vi "Triggers-Start.vi"(7 "Setup/Logging queue element":T1={"Imaging Protocol"=enum."Live Imaging", "Number of Trials"=0, "Frame Size"=512, "# Averaged frames"=0, "Dwell time (us)"=0.0, "Index of Z-plane"=0, "Timelapse?"=FALSE, "Logging process is active"=FALSE, "Speed logging enabled"=FALSE, "tdms file ref"=refnum, "path"=path "", "Trial Number"=0, "Expected # points acquired"=FALSE, "Manually stopped"=FALSE, "Ch0 data"=[], "Ch1 data"=[], "Last trial"=FALSE, "Points acquired"={"Ch0 last trial"=0, "Ch1 last trial"=0, "All trials"=0}} {"Frame Size" items=["100X100"=100, "128X128"=128, "200X200"=200, "256X256"=256, "512X512"=512, "1024x1024"=1024, "2048x2048"=2048]; "Dwell time (us)" format="%#.6g"}, 8 "error in (no error)":errorcluster, 11 "FPGA Ref":T5) -> (0 "error out":errorcluster)   [LabVIEW 2013]
uses:
  RIG-SPECIFIC FILES/FPGA Refs/FPGA Ref.ctl
  Typedefs/Logging queue element.ctl
  Typedefs/Imaging Protocols enum.ctl
  Typedefs/Frame Size.ctl
  Typedefs/Acquired points count.ctl
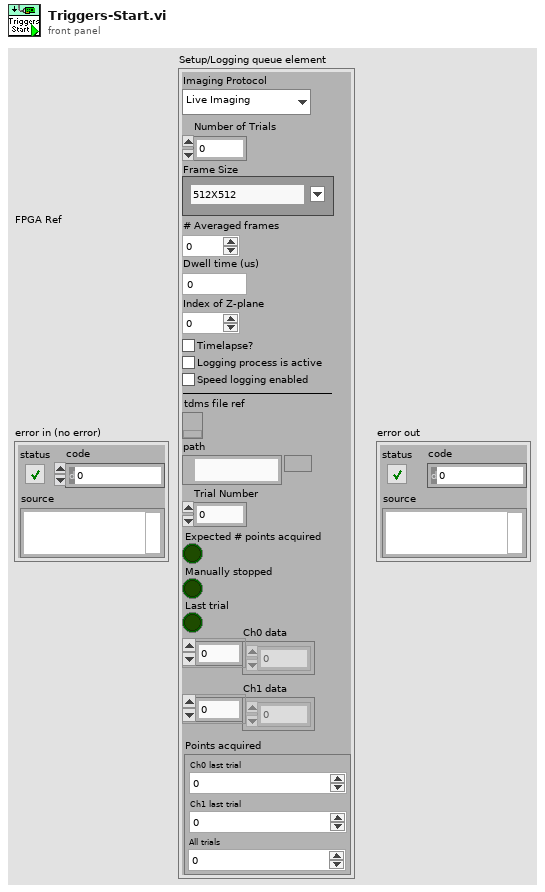
[diagram p1: front panel]
types:
  T1 = typedef "Logging queue element.ctl" = cluster{"Imaging Protocol":T2, "Number of Trials":u16, "Frame Size":T3, "# Averaged frames":u16, "Dwell time (us)":dbl, "Index of Z-plane":i32, "Timelapse?":bool, "Logging process is active":bool, "Speed logging enabled":bool, "tdms file ref":refnum<k34>, "path":path, "Trial Number":i32, "Expected # points acquired":bool, "Manually stopped":bool, "Ch0 data":u32[], "Ch1 data":u32[], "Last trial":bool, "Points acquired":T4}
  T2 = typedef "Imaging Protocols enum.ctl" = enum16{"AOL Z-Stack", "Motor Z Stack", "Functional Acquisition", "Single Plane Acquisition", "Volume Acquisition", "Live Imaging", "Live Plane Imaging", "Live Volume Imaging"}
  T3 = typedef "Frame Size.ctl" = u16
  T4 = typedef "Acquired points count.ctl" = cluster{"Ch0 last trial":u64, "Ch1 last trial":u64, "All trials":u64}
  T5 = typedef "FPGA Ref.ctl" = refnum<k20>
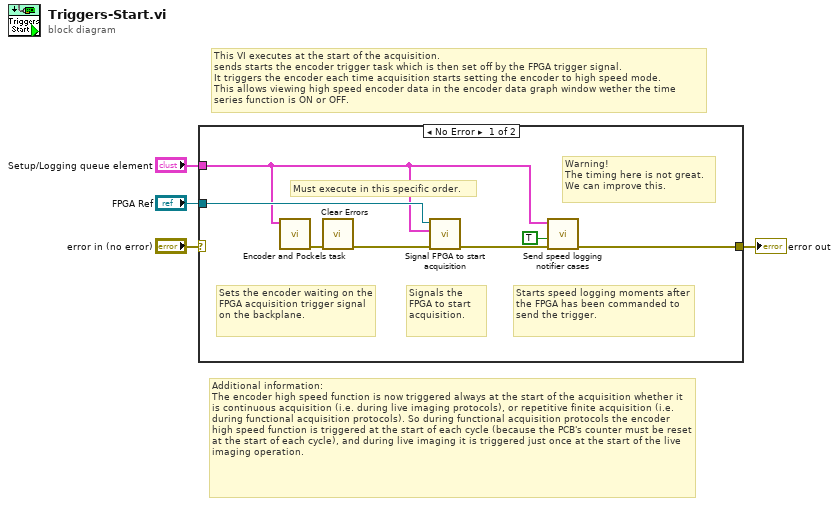
[diagram p0: block diagram]
diagram:
  # "Additional information:\nThe encoder high speed function is now triggered always at the start of the acquisition whether it is continuous acquisition (i.e. during live imaging protocols), or repetitive finite acquisition (i.e. during functional acquisition protocols). So during functional acquisition protocols the encoder high speed function is triggered at the start of each cycle (because the PCB's counter must be reset at the start of each cycle), and during live imaging it is triggered just once at the start of the live imaging operation."
  # "This VI executes at the start of the acquisition.\nsends starts the encoder trigger task which is then set off by the FPGA trigger signal.\nIt triggers the encoder each time acquisition starts setting the encoder to high speed mode.\nThis allows viewing high speed encoder data in the encoder data graph window wether the time series function is ON or OFF."
  n1 = case shown="No Error" "error in (no error)" {
    selector: "error in (no error)" -> [_ w12]
    tunnel: "FPGA Ref" -> [w11 _]
    tunnel: [w7 w12] -> w3
    tunnel: "Setup/Logging queue element" -> [w6 _]
    frame No Error {
      # "Warning!\nThe timing here is not great.\nWe can improve this."
      # "Starts speed logging moments after the FPGA has been commanded to send the trigger."
      # "Signals the FPGA to start acquisition."
      # "Sets the encoder waiting on the FPGA acquisition trigger signal on the backplane."
      # "Must execute in this specific order."
      n2 = call "Encoder and Pockels task.vi"("Setup/Logging queue element"=w6) -> ("error out"=w10:errorcluster)  [unwired: 10 in]
      n3 = call <vilib>:"Clear Errors.vi"("error in (no error)"=w10) -> ("error out"=w5:errorcluster)  [unwired: 6 in]
      n4 = call "Signal FPGA to start acquisition.vi"("error in (no error)"=w5, "Logging queue element"=w6, "FPGA VI Ref"=w11) -> ("error out"=w8:errorcluster)  [unwired: 8 in]
      n5 = call "Send speed logging notifier cases.vi"("error in"=w8, "Log speed data = T (Unused)"=TRUE ("Log speed data"), "Setup/Logging queue element"=w6) -> ("error out"=w7:errorcluster)  [unwired: 8 in]
    }
    frame Error {
    }
  }
  "error out" <- w3
